vi "Field Relative Swerve.vi"(8 "Field Relative Active":bool, 11 "Axes Magnitudes":cluster{"X":dbl, "Y":dbl, "Z":dbl}) -> (3 "Axes Mag. Changed":cluster{"X":dbl, "Y":dbl, "Z":dbl})   [LabVIEW 2016, in "Huskie Swerve.lvlib"]
uses:
  Huskie Swerve.lvlib
  Refname/Sensors.ctl
  Refname/Refname to String (Sensors).vi
  <vilib>/Rock Robotics/WPI/ThirdParty/Sensors/ADIS16448 IMU/ADIS16448_IMU.lvlib
  <vilib>/ptbypt/NI_PtbyPt.lvlib
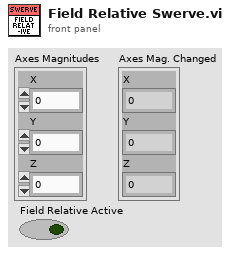
[diagram p1: front panel]
types:
  T1 = typedef "Huskie Swerve.lvlib/Sensors.ctl" = enum16{"Gyro", "Vision USB", "Button Pressed", "Other sensor", "Generic Sensor"}
  T2 = typedef "ADIS16448_IMU.lvlib/ADI_IMU_ADIS16448_InterruptDevRef.ctl" = cluster{"ADI IMU DevRef":T3, "InterruptRef":T5}
  T3 = typedef "ADIS16448_IMU.lvlib/ADI_IMU_ADIS16448_IMUDevRef.ctl" = cluster{"DevStatus":errorcluster, "Handle":i32, "SPI Bus":T4, "Device Found":bool, "Device Ready":bool, "Yaw Axis":enum16{"X", "Y", "Z"}, "AHRS Algorithm":enum16{"Complementary", "Madgwick"}, "Serial":u16, "Lot ID 2":u16, "Lot ID 1":u16, "Product ID":u16}
  T4 = typedef "spi_bus.ctl" = enum16{"SPI On-Board, CS0", "SPI On-Board, CS1", "SPI On-Board, CS2", "SPI On-Board, CS3", "SPI MXP", "Invalid"}
  T5 = typedef "WPI_InterruptRef.ctl" = cluster{"DevStatus":errorcluster, "InterruptIndex":T6}
  T6 = typedef "FPGA_InterruptIndex.ctl" = enum8{"0", "1", "2", "3", "4", "5", "6", "7", "Invalid"}
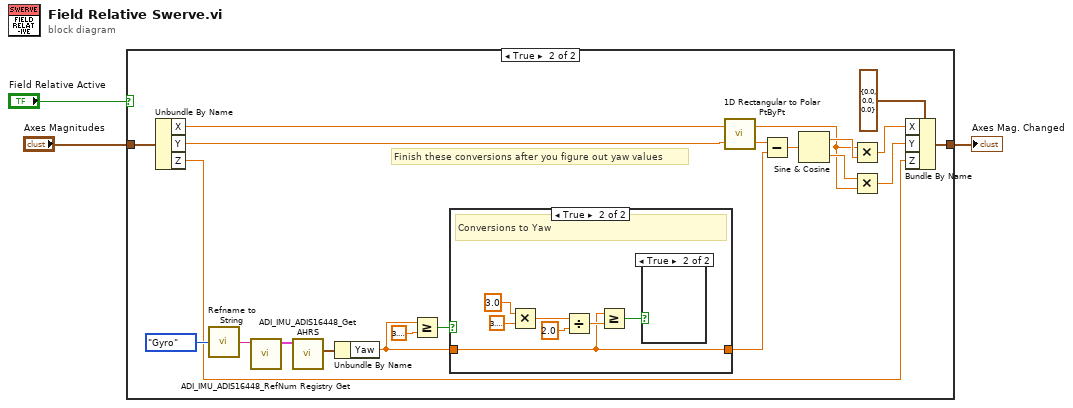
[diagram p0: block diagram]
diagram:
  n1 = case shown="True" "Field Relative Active" {
    tunnel: "Axes Magnitudes" -> [w4 w21]
    tunnel: [w4 w5] -> w2
    frame False {
    }
    frame True {
      # "Finish these conversions after you figure out yaw values"
      n2 = Unbundle By Name(w21) -> ("X"=w20:dbl, "Y"=w19:dbl, "Z"=w6:dbl)
      n3 = call-poly "Refname to String.vi"("Enum"=Sensors."Gyro") -> ("resulting string"=w24:string)
      n4 = call <vilib>:"ADI_IMU_ADIS16448_RefNum Registry Get.vi"("refnum name"=w24) -> ("ADI IMU Interrupt DevRef"=w22:T2)  [unwired: 9 in, 1 out]
      n5 = call <vilib>:"ADI_IMU_ADIS16448_Get AHRS.vi"("ADI IMU Interrupt DevRef"=w22) -> ("IMU AHRS Out"=w23:cluster{"Pitch":dbl, "Roll":dbl, "Yaw":dbl})  [unwired: 6 in, 4 out]
      n6 = Unbundle By Name(w23) -> ("Yaw"=w15:dbl)
      n7 = Greater Or Equal?(x=w15, y=3.141592653589793) -> (x >= y?=w16:bool)
      n8 = case shown="True" w16 {
        tunnel: w15 -> [w26 w28]
        tunnel: [w26 w28] -> w14
        frame False {
        }
        frame True {
          # "Conversions to Yaw"
          n9 = Multiply(x=3.0, y=3.141592653589793) -> (x*y=w31:dbl)
          n10 = Divide(x=w31, y=2.0) -> (x/y=w29:dbl)
          n11 = Greater Or Equal?(x=w28, y=w29) -> (x >= y?=w27:bool)
          n12 = case shown="True" w27 {
            frame False {
            }
            frame True {
            }
          }
        }
      }
      n13 = call <vilib>:"1D Rectangular to Polar PtByPt.vi"("y"=w19, "x"=w20) -> ("phase"=w18:dbl, "magnitude"=w10:dbl)
      n14 = Subtract(x=w18, y=w14) -> (x-y=w13:dbl)
      n15 = Sine & Cosine(0:w13) -> (1:w12:dbl, 2:w11:dbl)
      n16 = Multiply(x=w10, y=w12) -> (x*y=w8:dbl)
      n17 = Multiply(x=w11, y=w10) -> (x*y=w7:dbl)
      n18 = Bundle By Name(cluster=cluster{"X":dbl, "Y":dbl, "Z":dbl} {"X"=0.0, "Y"=0.0, "Z"=0.0} ("Axes Magnitudes 3"), "X"=w8, "Y"=w7, "Z"=w6) -> (w5:cluster{"X":dbl, "Y":dbl, "Z":dbl})
    }
  }
  "Axes Mag. Changed" <- w2
